vi "Construct SQL.vi"(6 "Time Bucket":T1, 7 "max points":i32=1 min=1, 8 "error in (no error)":errorcluster, 10 "PG path":string, 11 "Database Viewer":refnum<class "Database Viewer.lvclass">) -> (0 "error out":errorcluster, 2 "SQL string":string, 3 "Database Viewer out":refnum<class "Database Viewer.lvclass">)   [LabVIEW 2019, in "Database Viewer.lvclass"]
uses:
  Database Viewer.lvclass
  typedefs/Time Bucket--enum.ctl
  Database Viewer.lvclass/Database Viewer.ctl
  <userlib>/LevyLab/LV-Data/LV-Data.PG/LV-Data.PGSQL.lvclass
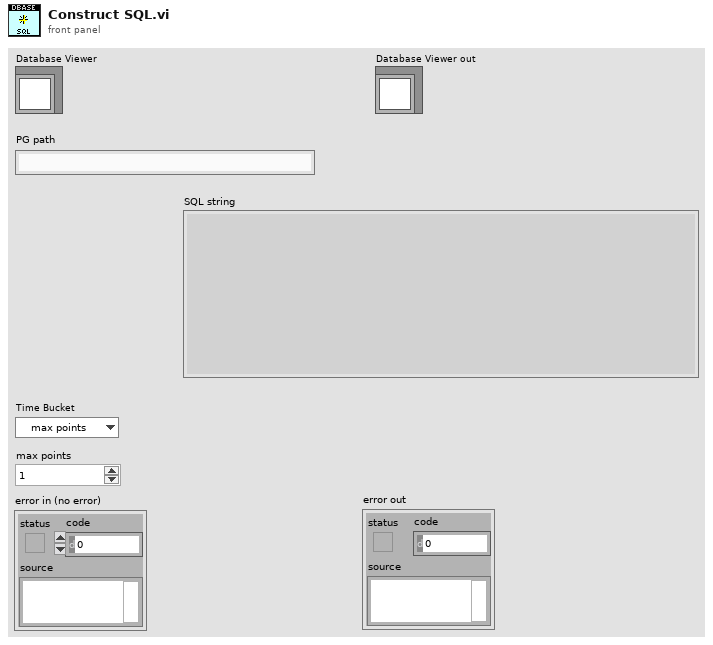
[diagram p1: front panel]
types:
  T1 = typedef "Database Viewer.lvclass/Time Bucket--enum.ctl" = enum16{"max points", "automatic", "1 second", "10 seconds", "1 minute", "10 minutes", "1 hour", "10 hours", "1 day", "10 days"}
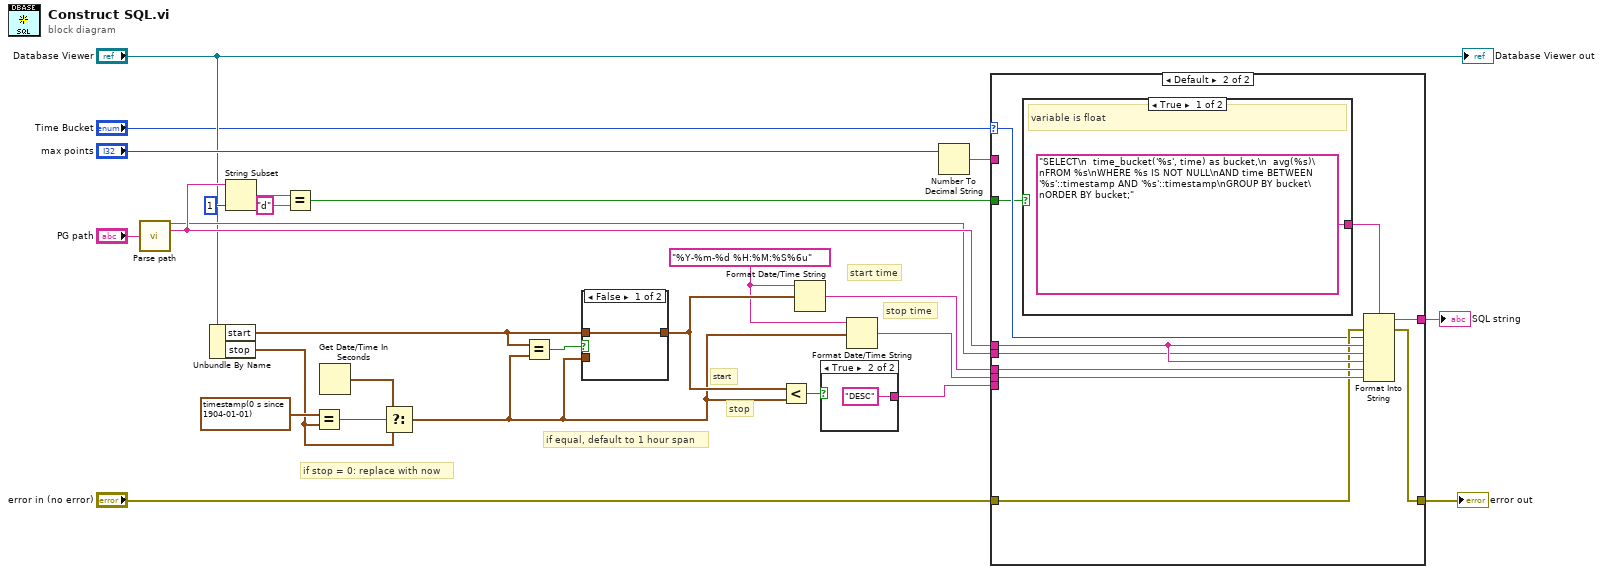
[diagram p0: block diagram]
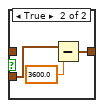
[diagram p2: hidden frame]
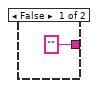
[diagram p3: hidden frame]
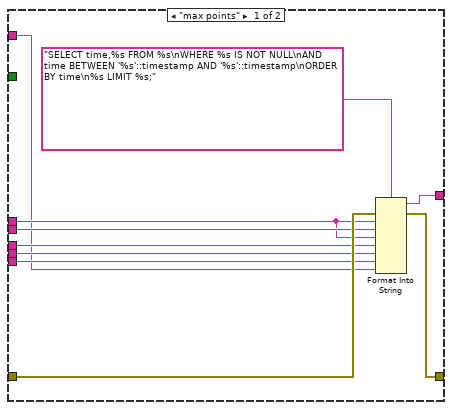
[diagram p4: hidden frame]
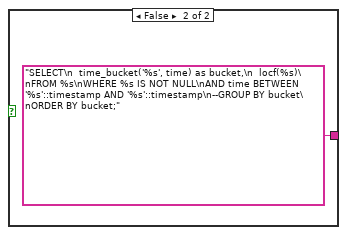
[diagram p5: hidden frame]
diagram:
  w18 = "%Y-%m-%d %H:%M:%S%6u" ("time format string (%c)")
  # "stop time"
  # "if equal, default to 1 hour span"
  # "if stop = 0: replace with now"
  # "stop"
  # "start"
  # "start time"
  n1 = call <userlib>:"Parse path.vi"("PG Path"="PG path") -> ("Table path"=w11:string, "Column path"=w12:string)  [unwired: 10 in, 3 out]
  n2 = Unbundle By Name("Database Viewer") -> ("start"=w7:timestamp, "stop"=w6:timestamp)
  n3 = String Subset(string=w12, length (rest)=1 ("length (rest)")) -> (substring=w21:string)  [unwired: 1 in]
  n4 = Equal?(x=w21, y="d") -> (x = y?=w3:bool)
  n5 = Equal?(x=timestamp(0 s since 1904-01-01) ("stop timestamp"), y=w6) -> (x = y?=w25:bool)
  n6 = Get Date/Time In Seconds() -> (seconds since 1Jan1904=w23:timestamp)
  n7 = Select(t=w23, s=w25, f=w6) -> (s? t:f=w4:timestamp)
  n8 = Equal?(x=w7, y=w4) -> (x = y?=w5:bool)
  n9 = case shown="False" w5 {
    tunnel: [w28 w29] -> w19
    tunnel: w7 -> [w28 _]
    tunnel: w4 -> [_ w30]
    frame False {
    }
    frame True {
      n10 = Subtract(x=w30, y=3600.0) -> (x-y=w29:timestamp)
    }
  }
  n11 = Less?(x=w19, y=w4) -> (x < y?=w27:bool)
  n12 = Format Date/Time String(time format string (%c)=w18, seconds (now)=w19) -> (date/time string=w9:string)  [unwired: 1 in]
  n13 = case shown="True" w27 {
    tunnel: ["" "DESC"] -> w13
    frame False {
    }
    frame True {
    }
  }
  n14 = Format Date/Time String(time format string (%c)=w18, seconds (now)=w4) -> (date/time string=w10:string)  [unwired: 1 in]
  n15 = Number To Decimal String(number="max points") -> (decimal integer string=w14:string)  [unwired: 1 in]
  n16 = case shown="Default" "Time Bucket" {
    selector: "Time Bucket" -> [_ w45]
    tunnel: w12 -> [w39 w53]
    tunnel: w11 -> [w40 w52]
    tunnel: w10 -> [w37 w51]
    tunnel: w9 -> [w38 w50]
    tunnel: "error in (no error)" -> [w42 w47]
    tunnel: [w41 w49] -> w16
    tunnel: [w36 w48] -> w15
    tunnel: w14 -> [w34 _]
    tunnel: w13 -> [w35 _]
    tunnel: w3 -> [_ w44]
    frame "max points" {
      n17 = Format Into String(format string="SELECT time,%s FROM %s\nWHERE %s IS NOT NULL\nAND time BETWEEN '%s'::timestamp AND '%s'::timestamp\nORDER BY time\n%s LIMIT %s;", error in=w42, w39, w40, w39, w38, w37, w35, w34) -> (resulting string=w36:string, error out=w41:errorcluster)  [unwired: 1 in]
    }
    frame Default {
      n18 = case shown="True" w44 {
        tunnel: ["SELECT\n  time_bucket('%s', time) as bucket,\n  avg(%s)\nFROM %s\nWHERE %s IS NOT NULL\nAND time BETWEEN '%s'::timestamp AND '%s'::timestamp\nGROUP BY bucket\nORDER BY bucket;" ("format string") "SELECT\n  time_bucket('%s', time) as bucket,\n  locf(%s)\nFROM %s\nWHERE %s IS NOT NULL\nAND time BETWEEN '%s'::timestamp AND '%s'::timestamp\n--GROUP BY bucket\nORDER BY bucket;" ("format string")] -> w46
        frame True {
          # "variable is float"
        }
        frame False {
        }
      }
      n19 = Format Into String(format string=w46, error in=w47, w45, w53, w52, w53, w50, w51) -> (resulting string=w48:string, error out=w49:errorcluster)  [unwired: 1 in]
    }
  }
  "SQL string" <- w15
  "error out" <- w16
  "Database Viewer out" <- "Database Viewer"
